vi "Light Grayscale.vi"() -> ()   [LabVIEW 2014]
doc: "This example illustrates the use of Light Meter VIs to perform intensity measurements on regions of an image. The sequence of images in this example represents an infrared view of an electronic device under test. The VI performs an intensity measurement on a rectangular area of the image to detect the overheat of a specific component."
uses:
  <vilib>/vision/NI_Vision_Development_Module.lvlib
panel:
  out "Image #:":i32
  out "Histogram Report":T1 {"Standard  Variation" format="%.2f"; "Mean Value" format="%.2f"; "Interval Width" format="%.2f"; "Starting Value" format="%.2f"; "Maximal Value" format="%.2f"; "Minimal Value" format="%.2f"}
  in  "Delay(ms)":u32(slide)=918 scale=0.0..3000.0
  out "Region Report":T2 {"Mean Value" format="%#_4g"; "Standard Variation" format="%#_4g"; "Minimal Value" format="%#_4g"; "Maximal Value" format="%#_4g"; "Area (calibrated)" format="%#_4g"; "Area (pixels)" format="%.4f"; "%" format="%#_4g"}
  out "Intensity Chart":sgl(graph)
  out "Image":T3(plugin-control)
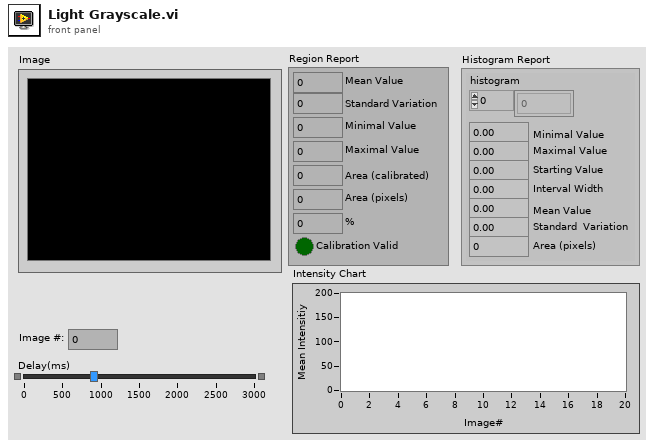
[diagram p1: front panel]
types:
  T1 = cluster{"histogram":u32[], "Minimal Value":sgl, "Maximal Value":sgl, "Starting Value":sgl, "Interval Width":sgl, "Mean Value":sgl, "Standard  Variation":sgl, "Area (pixels)":i32}
  T2 = cluster{"Mean Value":sgl, "Standard Variation":sgl, "Minimal Value":sgl, "Maximal Value":sgl, "Area (calibrated)":sgl, "Area (pixels)":u32, "%":sgl, "Calibration Valid":bool}
  T3 = typedef "IMAQ Image.ctl" = refnum<image>
  T4 = typedef "Image Type" = u32
  T5 = typedef "IMAQ Rectangle" = cluster{"Left":i32, "Top":i32, "Right":i32, "Bottom":i32, "Rotation":dbl}
  T6 = typedef "ROI Descriptor" = cluster{"Global Rectangle":i32[], "Contours":cluster{"ID":enum32{"External", "Internal"}, "Type":u32, "Coordinates":i32[]}[]}
  T7 = cluster{"Mean Value":sgl, "Standard Variation":sgl, "Minimal Value":sgl, "Maximal Value":sgl, "Area (calibrated)":sgl, "Area (pixels)":u32, "%":sgl, "Calibration Valid":bool}[]
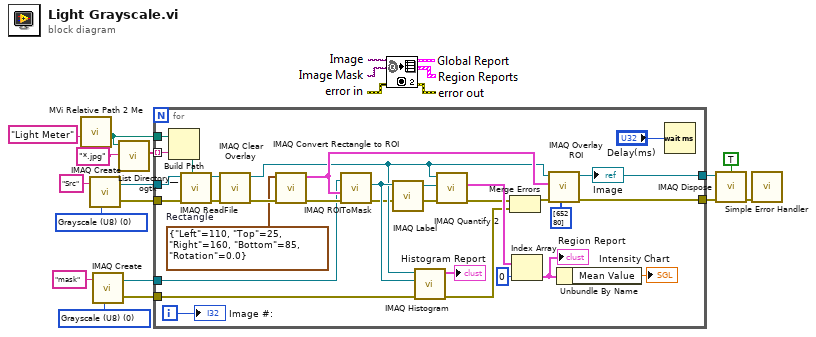
[diagram p0: block diagram]
diagram:
  w4 = T4 0 items=["Grayscale (U8)", "Grayscale (I16)", "Grayscale (SGL)", "Complex (CSG)", "RGB (U32)", "HSL (U32)", "RGB (U64)", "Grayscale (U16)"] ("Image Type")
  w12 = T4 0 items=["Grayscale (U8)", "Grayscale (I16)", "Grayscale (SGL)", "Complex (CSG)", "RGB (U32)", "HSL (U32)", "RGB (U64)", "Grayscale (U16)"] ("Image Type")
  n1 = call "MVi Relative Path 2 Me.vi"("Relative Path"="Light Meter") -> ("Appended Dir"=w8:path)  [unwired: 5 in, 1 out]
  n2 = call "IMAQ Create"("Image Name"="Src" ("name or relative path"), "Image Type"=w12) -> ("New Image"=w9:T3, "error out"=w10:errorcluster)  [unwired: 2 in, 1 out]
  n3 = call "IMAQ Create"("Image Name"="mask" ("name or relative path"), "Image Type"=w4) -> ("New Image"=w3:T3, "error out"=w1:errorcluster)  [unwired: 2 in, 1 out]
  n4 = call "List Directory__ogtk.vi"("pattern"="*.jpg", "directory path"=w8) -> ("file names"=w6:string[])  [unwired: 2 in, 3 out]
  n5 = for {
    tunnel: w8 -> [w45]
    tunnel: [w32] -> w15
    tunnel: [w34] -> w14
    tunnel: w10 -> [w46]
    tunnel: w9 -> [w42]
    tunnel: w6 -> [w44] mode=indexing
    tunnel: w3 -> [w31]
    tunnel: w1 -> [w19]
    i -> [w17]
    w37 = T5 {"Left"=110, "Top"=25, "Right"=160, "Bottom"=85, "Rotation"=0.0}  # Rectangle
    n6 = Build Path(base path=w45, name or relative path=w44) -> (appended path=w43:path)
    n7 = call "IMAQ ReadFile"("File Path"=w43, "error in (no error)"=w46, "Image"=w42) -> ("error out"=w41:errorcluster, "Image Out"=w40:T3)  [unwired: 4 in, 3 out]
    n8 = call "IMAQ Clear Overlay"("error in (no error)"=w41, "Image"=w40) -> ("error out"=w38:errorcluster, "Image Out"=w25:T3)  [unwired: 1 in, 7 out]
    n9 = call "IMAQ Convert Rectangle to ROI"("error in (no error)"=w38, "Rectangle"=w37) -> ("error out"=w36:errorcluster, "ROI Descriptor"=w35:T6)  [unwired: 7 out]
    n10 = call "IMAQ ROIToMask"("error in (no error)"=w36, "ROI Descriptor"=w35, "Image"=w31) -> ("error out"=w18:errorcluster, "Image Out"=w26:T3)  [unwired: 2 in, 2 out]
    n11 = call "IMAQ Label"("error in (no error)"=w18, "Image Src"=w26) -> ("error out"=w27:errorcluster, "Image Dst Out"=w28:T3)  [unwired: 2 in, 1 out]
    n12 = call "IMAQ Histogram"("error in (no error)"=w19, "Image Mask"=w26, "Image"=w25) -> ("error out"=w21:errorcluster, "Histogram Report"=→"Histogram Report":T1)  [unwired: 7 in]
    n13 = call "IMAQ Quantify 2"("error in (no error)"=w27, "Image Mask"=w28, "Image"=w25) -> ("error out"=w22:errorcluster, "Region Reports"=w30:T7)  [unwired: 6 in, 1 out]
    n14 = Merge Errors(w22, w21) -> (w23:errorcluster)
    n15 = Index Array(array=w30, index=0) -> (element=w29:T2)
    "Region Report" <- w29
    n16 = call "IMAQ Overlay ROI"("Colors (Green)"=u32[] [65280] ("Colors (Red)"), "error in (no error)"=w23, "ROI Descriptor"=w35, "Image"=w25) -> ("error out"=w34:errorcluster, "Image Out"=w32:T3)  [unwired: 2 in, 4 out]
    "Image" <- w32
    n17 = Unbundle By Name(w29) -> ("Mean Value"=→"Intensity Chart":sgl)
    n18 = Wait (ms)(milliseconds to wait="Delay(ms)") -> ()  [unwired: 1 out]
    "Image #:" <- w17
  }
  n19 = call "IMAQ Dispose"("All Images? (No)"=TRUE, "Image"=w15, "error in (no error)"=w14) -> ("error out"=w16:errorcluster)  [unwired: 3 out]
  n20 = call <vilib>:"Simple Error Handler.vi"("error in (no error)"=w16) -> ()  [unwired: 4 in, 5 out]
